vi "LEIN CMD read STAT.vi"(7 "CMD":T1={"SID"=0, "ANF"=FALSE, "CMD"=enum."TASK", "DATA"=[]}, 11 "error in (no error)":errorcluster) -> (4 "SID":u8, 6 "Data":u8[](array[numeric]), 8 "STAT ID":u8, 10 "STAT Part":u8, 14 "ACK":bool, 15 "error out":errorcluster)   [LabVIEW 2011]
uses:
  Defenitions/LEIN CMD Cluster.ctl
  Defenitions/LEIN CMD List.ctl
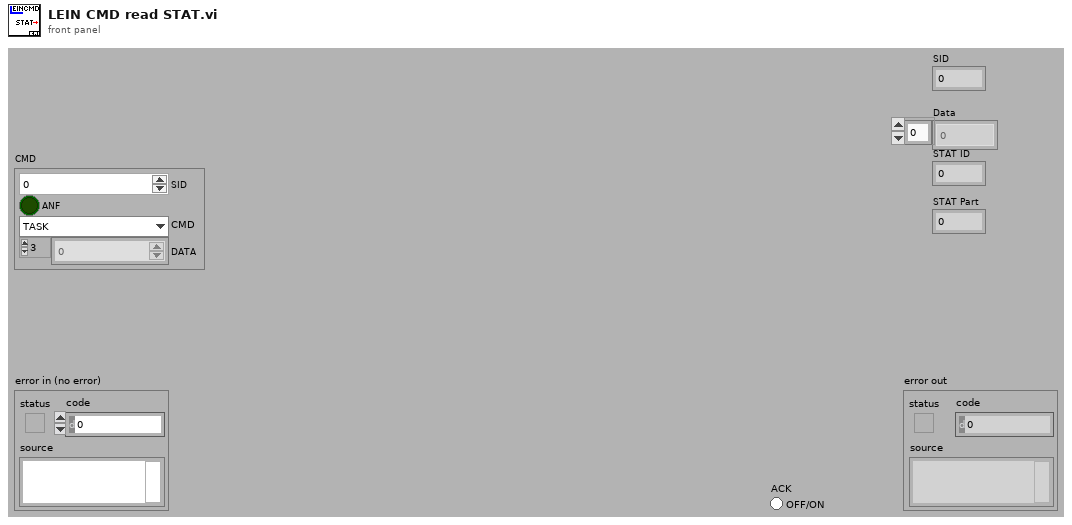
[diagram p1: front panel]
types:
  T1 = typedef "LEIN CMD Cluster.ctl" = cluster{"SID":u8, "ANF":bool, "CMD":T2, "DATA":u8[]}
  T2 = typedef "LEIN CMD List.ctl" = enum8{"ACTI", "TASK", "RES0", "STAT", "RES1", "RES2", "RES3", "USER"}
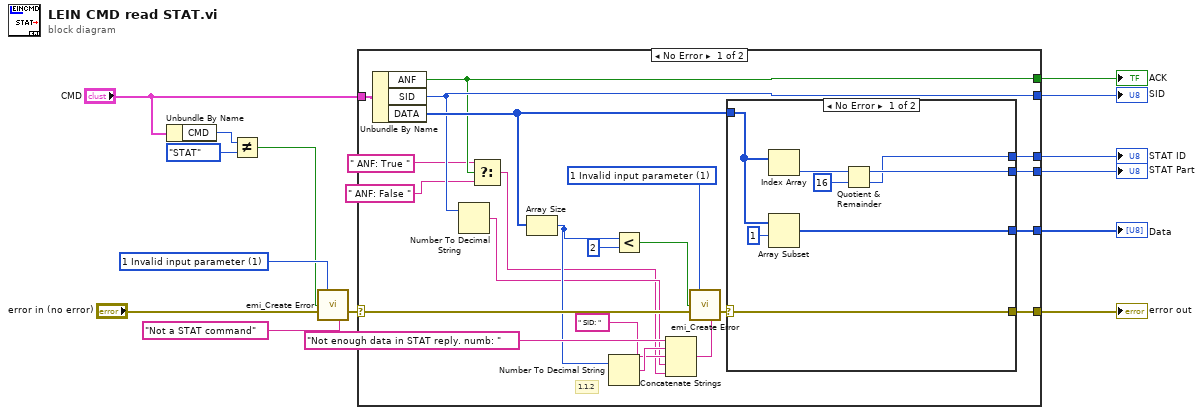
[diagram p0: block diagram]
diagram:
  w14 = 1 items=["0 No Error"=0, "1 Invalid input parameter"=1, "6 Generic file IO "=6, "7 File not Found"=7, "35 Generic Pring Error"=35, "37 Device not Found"=37, "39 Device Unit Error"=39, "40 Could fot Open Device"=40, "42 Generic Error"=42, "52 Unknown Message"=52, "98 Bad File type"=98, "99 Bad File Version"=99, "100 Bad Data in File"=100, "1018 Unspecefied Error"=1018, "1041 Incorrect Password"=1041, "1043 Feature not in this version"=1043, "1109 Unsuported Data type"=1109, "1444 Did not close sucessfully"=1444] ("Error Code")
  n1 = Unbundle By Name("CMD") -> ("CMD"=w9:T2)
  n2 = Not Equal?(x=w9, y=LEIN_CMD_List."STAT") -> (x != y?=w7:bool)
  n3 = call "emi_Create Error.vi"("Error Code"=w14, "Error(T)"=w7, "error in (no error)"="error in (no error)", "Append String(\"\")"="Not a STAT command" ("Append String(\"\")")) -> ("error out"=w10:errorcluster)  [unwired: 11 in]
  n4 = case shown="No Error" w10 {
    selector: w10 -> [w34 w46]
    tunnel: [w27 w46] -> w11
    tunnel: "CMD" -> [w36 _]
    tunnel: [w21 _] -> w5
    tunnel: [w18 _] -> w4
    tunnel: [w30 _] -> w3
    tunnel: [w29 _] -> w2
    tunnel: [w28 _] -> w1
    frame No Error {
      w32 = 1 items=["0 No Error"=0, "1 Invalid input parameter"=1, "6 Generic file IO "=6, "7 File not Found"=7, "35 Generic Pring Error"=35, "37 Device not Found"=37, "39 Device Unit Error"=39, "40 Could fot Open Device"=40, "42 Generic Error"=42, "52 Unknown Message"=52, "98 Bad File type"=98, "99 Bad File Version"=99, "100 Bad Data in File"=100, "1018 Unspecefied Error"=1018, "1041 Incorrect Password"=1041, "1043 Feature not in this version"=1043, "1109 Unsuported Data type"=1109, "1444 Did not close sucessfully"=1444] ("Error Code")
      # "1.1.2"
      n5 = Unbundle By Name(w36) -> ("ANF"=w18:bool, "SID"=w21:u8, "DATA"=w31:u8[])
      n6 = Number To Decimal String(number=w21) -> (decimal integer string=w19:string)  [unwired: 1 in]
      n7 = Select(t=" ANF: True " ("string"), s=w18, f=" ANF: False " ("string")) -> (s? t:f=w15:string)
      n8 = Array Size(array=w31) -> (size(s)=w23:i32)
      n9 = Number To Decimal String(number=w23) -> (decimal integer string=w22:string)  [unwired: 1 in]
      n10 = Less?(x=w23, y=2) -> (x < y?=w33:bool)
      n11 = Concatenate Strings("Not enough data in STAT reply. numb: " ("Source String(\"\")"), w22, " SID: " ("string"), w19, w15) -> (w24:string)
      n12 = call "emi_Create Error.vi"("Error Code"=w32, "Error(T)"=w33, "error in (no error)"=w34, "Append String(\"\")"=w24) -> ("error out"=w26:errorcluster)  [unwired: 11 in]
      n13 = case shown="No Error" w26 {
        selector: w26 -> [w37 w45]
        tunnel: w31 -> [w40 _]
        tunnel: [w42 _] -> w30
        tunnel: [w41 _] -> w29
        tunnel: [w38 _] -> w28
        tunnel: [w37 w45] -> w27
        frame No Error {
          n14 = Index Array(array=w40) -> (element=w43:u8)  [unwired: 1 in]
          n15 = Array Subset(array=w40, index=1) -> (w38:u8[])  [unwired: 1 in]
          n16 = Quotient & Remainder(x=w43, y=u8 16) -> (x-y*floor(x/y)=w42:u8, floor(x/y)=w41:u8)
        }
        frame Error {
        }
      }
    }
    frame Error {
    }
  }
  "error out" <- w11
  "SID" <- w5
  "STAT ID" <- w2
  "STAT Part" <- w3
  "ACK" <- w4
  "Data" <- w1
